vi "_Read.vi"(8 "error in (no error)":errorcluster, 10 "Count":i32, 11 "Stream in":refnum<class "Stream.lvclass">) -> (0 "error out":errorcluster, 2 "Data":string, 3 "Stream out":refnum<class "Stream.lvclass">)   [LabVIEW 2020, in "Stream.lvlib" / "Stream.lvclass"]
uses:
  Stream.lvclass
  <vilib>/Utility/error.llb/Error Cluster From Error Code.vi
  <vilib>/ErrorRing/Error Ring.xnode
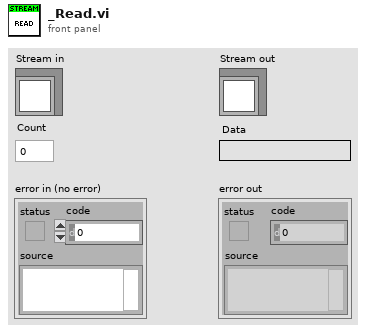
[diagram p1: front panel]
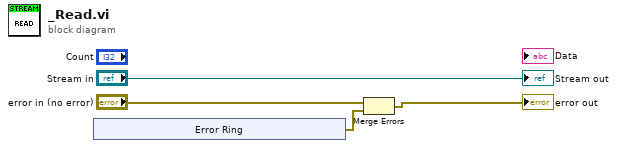
[diagram p0: block diagram]
diagram:
  n1 = xnode "Error Ring"() -> ("error out"=w3:errorcluster)
  n2 = Merge Errors("error in (no error)", w3) -> (→"error out":errorcluster)
  "Stream out" <- "Stream in"
